vi "ATCcont.vi"() -> ()   [LabVIEW 2014]
doc: "ATC app"
panel:
  in  "정지":bool
  in  "피드백":bool
  in  "정보1":bool
  in  "도움말":bool
  in  "?":bool
  in  "?":bool
  in  "탭":T1(tab)
  in  "메모":string="필요한 메모를 할수 있습니다. "
  in  "SID&RadarVector. 2":string="SID&RadarVector. "
  in  "인사말":string="인사말"
  in  "CD관제기관":string="관제기관"
  in  "콜사인":string="콜사인\n콜사인\n콜사인"
  in  "도착공항":string="도착공항"
  in  "SID&RadarVector":string="SID&RadarVector"
  in  "비행고도":string="비행고도"
  in  "인사말2":string="인사말"
  in  "콜사인2":string="콜사인"
  in  "콜사인3":string="콜사인"
  in  "콜사인4":string="콜사인"
  in  "콜사인5":string="콜사인"
  in  "콜사인6":string="콜사인"
  in  "도착공항2":string="도착공항"
  in  "제한고도":string="제한고도"
  in  "비행고도2":string="비행고도"
  in  "D접속주파수":string="접속주파수"
  in  "스콱번호":string="스콱번호"
  in  "도착공항3":string="도착공항"
  in  "SID&RadarVector. 3":string="SID&RadarVector. "
  in  "제한고도2":string="제한고도"
  in  "비행고도3":string="비행고도"
  in  "D접속주파수2":string="접속주파수"
  in  "스콱번호2":string="스쾃번호"
  in  "콜사인7":string="콜사인"
  in  "콜사인8":string="콜사인"
  in  "G관제기관":string="관제기관"
  in  "G접속주파수2":string="접속주파수"
  in  "G관제기관2":string="관제기관"
  in  "G접속주파수":string="접속주파수"
  in  "콜사인9":string="콜사인"
  in  "유도로 2":string="유도로"
  in  "유도로":string="유도로"
  in  "방향 2":string="방향"
  in  "방향":string="방향"
  in  "메모2":string="필요한 메모를 할수 있습니다. "
  in  "T관제기관2":string="관제기관"
  in  "콜사인24":string="콜사인"
  in  "T접속주파수2":string="접속주파수"
  in  "T접속주파수":string="접속주파수"
  in  "T관제기관":string="관제기관"
  in  "콜사인23":string="콜사인"
  in  "활주로9":string="활주로"
  in  "G관제기관4":string="관제기관"
  in  "콜사인22":string="콜사인"
  in  "콜사인21":string="콜사인"
  in  "콜사인20":string="콜사인"
  in  "콜사인19":string="콜사인"
  in  "활주로8":string="활주로"
  in  "활주로7":string="활주로"
  in  "콜사인17":string="콜사인"
  in  "활주로6":string="활주로"
  in  "콜사인18":string="콜사인"
  in  "활주로5":string="활주로"
  in  "콜사인16":string="콜사인"
  in  "활주로4":string="활주로"
  in  "콜사인15":string="콜사인"
  in  "활주로3":string="활주로"
  in  "콜사인14":string="콜사인"
  in  "콜사인13":string="콜사인"
  in  "현재기압2":string="현재기압"
  in  "출발공항":string="출발공항"
  in  "활주로2":string="활주로"
  in  "현재기압":string="현재기압"
  in  "출발공항2":string="출발공항"
  in  "활주로1":string="활주로"
  in  "콜사인12":string="콜사인"
  in  "콜사인11":string="콜사인"
  in  "G관제기관3":string="관제기관"
  in  "인사3":string="인사"
  in  "콜사인34 2":string="콜사인"
  in  "D관제기관2":string="관제기관"
  in  "D관제기관":string="관제기관"
  in  "T관제기관3":string="관제기관"
  in  "메모3":string="필요한 메모를 할수 있습니다. "
  in  "인사4":string="인사"
  in  "콜사인25":string="콜사인"
  in  "활주로10":string="활주로"
  in  "콜사인26":string="콜사인"
  in  "바람방향":string="바람방향"
  in  "풍속":string="풍속"
  in  "콜사인28":string="콜사인"
  in  "활주로13":string="활주로"
  in  "콜사인29":string="콜사인"
  in  "활주로12":string="활주로"
  in  "콜사인30":string="콜사인"
  in  "활주로14":string="활주로"
  in  "콜사인31":string="콜사인"
  in  "활주로15":string="활주로"
  in  "T관제기관4":string="관제기관"
  in  "콜사인32":string="콜사인"
  in  "현재고도":string="현재고도"
  in  "허가고도":string="허가고도"
  in  "콜사인33":string="콜사인"
  in  "접속주파수":string="접속주파수"
  in  "콜사인34":string="콜사인"
  in  "접속주파수2":string="접속주파수"
  in  "순항고도or이니셜고도":string="순항고도or이니셜고도"
  in  "D관제기관5":string="관제기관"
  in  "메모 4":string="필요한 메모를 할수 있습니다. "
  in  "인사5":string="인사"
  in  "D관제기관3":string="관제기관"
  in  "콜사인35":string="콜사인"
  in  "현재고도A":string="현재고도"
  in  "콜사인36":string="콜사인"
  in  "D관제기관4":string="관제기관"
  in  "허가고도4":string="허가고도"
  in  "허가고도5":string="허가고도"
  in  "콜사인37":string="콜사인"
  in  "콜사인38":string="콜사인"
  in  "허가고도6":string="허가고도"
  in  "허가고도7":string="허가고도"
  in  "콜사인39":string="콜사인"
  in  "콜사인40":string="콜사인"
  in  "C관제기관":string="관제기관"
  in  "A접속주파수":string="접속주파수"
  in  "C관제기관2":string="관제기관"
  in  "A접속주파수2":string="접속주파수"
  in  "콜사인41":string="콜사인"
  in  "콜사인38 2":string="콜사인"
  in  "D관제기관6":string="관제기관"
  in  "허가고도6 2":string="허가고도"
  in  "허가고도6 3":string="허가고도"
  in  "콜사인39 2":string="콜사인"
  in  "메모5":string="필요한 메모를 할수 있습니다. "
  in  "인사말 2":string="인사말"
  in  "허가고도 2":string="허가고도"
  in  "지점":string="지점"
  in  "허가고도7 2":string="허가고도"
  in  "콜사인38 3":string="콜사인"
  in  "콜사인39 3":string="콜사인"
  in  "허가고도7 3":string="허가고도"
  in  "지점 2":string="지점"
  in  "메모6":string="필요한 메모를 할수 있습니다. "
  in  "A관제기관3":string="관제기관"
  in  "콜사인46":string="콜사인"
  in  "날시정보":string="날시정보"
  in  "고도":string="고도"
  in  "콜사인47":string="콜사인"
  in  "A관제기관4":string="관제기관"
  in  "L활주로":string="활주로"
  in  "도착공항4":string="도착공항"
  in  "현재기압":string="현재기압"
  in  "콜사인48":string="콜사인"
  in  "A관제기관5":string="관제기관"
  in  "L활주로":string="활주로"
  in  "도착공항5":string="도착공항"
  in  "현재기압":string="현재기압"
  in  "콜사인49":string="콜사인"
  in  "고도":string="고도"
  in  "콜사인50":string="콜사인"
  in  "고도":string="고도"
  in  "콜사인51":string="콜사인"
  in  "고도":string="고도"
  in  "고도":string="고도"
  in  "콜사인52":string="콜사인"
  in  "콜사인53":string="콜사인"
  in  "A관제기관":string="관제기관"
  in  "풍속":string="풍속"
  in  "바람방향":string="바람방향"
  in  "L활주로3":string="활주로"
  in  "콜사인54":string="콜사인"
  in  "L활주로":string="활주로"
  in  "콜사인55":string="콜사인"
  in  "A관제기관2":string="관제기관"
  in  "L활주로":string="활주로"
  in  "ILS":string="주파수(ils)"
  in  "콜사인56":string="콜사인"
  in  "L활주로6":string="활주로"
  in  "ILS2":string="주파수(ils)"
  in  "콜사인57":string="콜사인"
  in  "T관제기관":string="관제기관"
  in  "T접속주파수":string="접속주파수"
  in  "콜사인58":string="콜사인"
  in  "콜사인59":string="콜사인"
  in  "관제기관":string="관제기관"
  in  "T접속주파수":string="접속주파수"
  in  "메모7":string="필요한 메모를 할수 있습니다. "
  in  "바람방향":string="바람방향"
  in  "관제기관":string="관제기관"
  in  "콜사인60":string="콜사인"
  in  "L활주로7":string="활주로"
  in  "콜사인61":string="콜사인"
  in  "풍속":string="풍속"
  in  "콜사인62":string="콜사인"
  in  "L활주로":string="활주로"
  in  "L활주로":string="활주로"
  in  "관제기관":string="관제기관"
  in  "콜사인63":string="콜사인"
  in  "관제기관3":string="관제기관"
  in  "콜사인64":string="콜사인"
  in  "L활주로":string="활주로"
  in  "G관제기관":string="관제기관"
  in  "G접속주파수":string="접속주파수"
  in  "콜사인65":string="콜사인"
  in  "관제기관":string="관제기관"
  in  "G접속주파수":string="접속주파수"
  in  "콜사인70":string="콜사인"
  in  "C활주로3":string="활주로"
  in  "C활주로2":string="활주로"
  in  "관제기관3 2":string="관제기관"
  in  "C활주로":string="활주로"
  in  "콜사인69":string="콜사인"
  in  "관제기관2":string="관제기관"
  in  "메모8":string="필요한 메모를 할수 있습니다. "
  in  "관제기관":string="관제기관"
  in  "콜사인66":string="콜사인"
  in  "콜사인67":string="콜사인"
  in  "게이트번호":string="게이트번호"
  in  "THEN":string="then"
  in  "콜사인68":string="콜사인"
  in  "게이트번호2":string="게이트번호"
  in  "THEN2":string="then"
  in  "콜사인10":string="콜사인"
  in  "관제기관4":string="관제기관"
  in  "콜사인71":string="콜사인"
  in  "콜사인72":string="콜사인"
  # "ver.3.0.0.55"
  # "~"
  # "Good"
  # "Clearance Delivery"
  # "Pilot"
  # "at FL"
  # "Request IFR Clearance to"
  # "Airport via"
  # "~"
  # "Good"
  # "Controller"
  # ",  Clearance  Delivery, standby."
  # "Pilot"
  # "Stand by,"
  # "Controller"
  # "Delivery 또는 Delivery, Are you ready to copy?"
  # "Pilot"
  # "Go Ahead 또는 Ready to copy"
  # "Airport via"
  # ", Cleared to"
  # "Controller"
  # "ft expect FL"
  # "then as filed. Climb and Maintain"
  # "Departure Frequency"
  # "Read back."
  # "Squawk"
  # "Pilot"
  # "Airport via"
  # "Cleared to"
  # ","
  # "then as filed."
  # "Climb and Maintain"
  # "ft expect FL"
  # "Departure Frequency"
  # "and  Squawk"
  # "Controller"
  # ", Read back is corrent contact"
  # "Ground"
  # "bye bye~."
  # "Pilot"
  # "Roger, contact"
  # ", bye bye~"
  # "Pilot"
  # "Good"
  # "~"
  # "ready for push back and Engine Start."
  # ","
  # ", Rwy"
  # "Push Back and Engine Start Approved, heading to"
  # "Controller"
  # ","
  # "QNH"
  # "Read Back."
  # "Pilot"
  # "Roger\nPush Back and Engine Start Approved, heading to"
  # ", Rwy"
  # "QNH"
  # "Ready for taxi to the Rwy"
  # ","
  # "Pilot"
  # "- Push back 완료 후 -"
  # ", Ready for Taxi to Rwy"
  # "Controller"
  # ", taxi to"
  # "via taxiway"
  # ", Roger"
  # "Pilot"
  # "via taxiway"
  # "Taxi to"
  # "- 활주로를 건널 상황일 때 -"
  # "Pilot"
  # "Request Cross Rwy"
  # "Controller"
  # ", cleared Cross Rwy"
  # "Pilot"
  # "cleared Cross Rwy"
  # "Controller"
  # "Squawk Mode C."
  # "Pilot"
  # ", Roger squawk mode 'C'"
  # "------------------------ 홀딩 포인트 도착 후 ----------------------------------"
  # "Pilot"
  # "hold short of Rwy"
  # ","
  # "Controller"
  # "Roger,"
  # "contact"
  # "Tower"
  # "bye bye~"
  # "Pilot"
  # "Contact"
  # "Pilot"
  # "Good"
  # "~"
  # ",  hold short Rwy"
  # ", Ready for Departure"
  # "(곧바로 이륙허가)"
  # "Controller"
  # ", wind"
  # "knot, cleared for take off."
  # "at"
  # "(활주로 정렬대기)"
  # "Controller"
  # "Line up and wait Rwy"
  # "Pilot"
  # "Line up and wait Rwy"
  # "Roger,"
  # "(홀딩 포인트에서 대기)"
  # "Controller"
  # ", Hold short rwy"
  # ","
  # "Pilot"
  # "Hold short of Rwy"
  # "Roger,"
  # "- 이 륙 후 -"
  # "Pilot"
  # "ft."
  # "Airborn Passing"
  # "ft, Climbing"
  # ","
  # "Controller"
  # ", contact"
  # "Departure,"
  # "bye bye~"
  # "Pilot"
  # ", Roger"
  # "Contact"
  # "Departure,"
  # "bye bye~"
  # "Good"
  # "~"
  # "Pilot"
  # "Passing"
  # "expect"
  # "with (SID)."
  # ","
  # ","
  # "Controller"
  # "Departure, Radar Contact, Climb via (SID) to"
  # ","
  # "."
  # "Pilot"
  # "Roger, Climb via"
  # ","
  # "-고도제한 해제시-"
  # "Controller"
  # "Departure, Radar Contact, Climb via (SID) to"
  # ", Cancel Level Restrictions."
  # "Pilot"
  # "Roger, Climb via (SID) to"
  # ", Cancel Level Restrictions,"
  # "-속도제한 해제시-"
  # "Controller"
  # "Departure, Radar Contact, Climb via (SID) to"
  # ", Cancel Speed Restrictions."
  # "Pilot"
  # "Roger, Climb via (SID) to"
  # ", Cancel Speed Restrictions,"
  # "Controller"
  # "Control,"
  # ", bye bye."
  # ", You are leaving my airspace, Contact"
  # "Pilot"
  # "Contact"
  # "G'day"
  # "Control,"
  # ","
  # "Pilot"
  # "Good"
  # "Decend and maintain FL"
  # "with (SID)."
  # "-하강 발부-"
  # "Controller"
  # "by"
  # ", Descend and Maintain"
  # "Pilot"
  # "Descend and Maintain"
  # "by"
  # "Pilot"
  # ","
  # "FL"
  # "with information"
  # ","
  # ", Expect vector to ILS Rwy"
  # "approach"
  # "Controller"
  # "QNH"
  # "Roger,"
  # "Pilot"
  # ", Expect vector to ILS Rwy"
  # "final approach"
  # "QNH"
  # "Controller"
  # ", Decend and maintain FL"
  # "Pilot"
  # "Decend and maintain FL"
  # "Roger,"
  # "Controller"
  # ", Decend and maintain"
  # "ft"
  # "Pilot"
  # "Roger"
  # "Decend and maintain"
  # "ft"
  # "Controller"
  # ","
  # "for landing"
  # "wind"
  # "knots active Rwy"
  # "at"
  # "Pilot"
  # "Roger,"
  # "Rwy"
  # "for landing"
  # "Controller"
  # ","
  # "approach use Rwy"
  # "ILS"
  # "Roger,"
  # "Pilot"
  # "Use Rwy"
  # "ILS"
  # "- 정 렬 후 -"
  # "Pilot"
  # "Approach,"
  # ", Established on Localizer."
  # "Controller"
  # "Tower,"
  # "Good day,"
  # "Roger, Contact"
  # "Pilot"
  # "Contact"
  # "Tower"
  # "Good day,"
  # "Pilot"
  # ","
  # "Inbound Approaching Rwy"
  # "Controller"
  # ", Wind"
  # "at"
  # "knots Rwy"
  # ", Cleared to land"
  # "Pilot"
  # "Rwy"
  # "Cleared to land"
  # "Pilot"
  # ","
  # "- 착 륙 후 -"
  # ","
  # "Pilot"
  # "Touch down with Rwy"
  # "Controller"
  # "Roger, change squawk mode Standby and contact"
  # "bye bye~"
  # "ground"
  # "Pilot"
  # ", Roger"
  # "bye bye~"
  # "Change squawk mode standby and contact"
  # "- 활주로를 건널 상황일 때 -"
  # "Pilot"
  # ","
  # "Request Cross Rwy"
  # "Controller"
  # ", Cross Rwy"
  # "approved."
  # "Pilot"
  # "Cross Rwy"
  # "approved"
  # ","
  # "Pilot"
  # "Ready to taxi to the Gate"
  # "Controller"
  # ", taxi to the gate"
  # "via taxi way"
  # "Roger,"
  # "Pilot"
  # "taxi to the gate"
  # "via taxi way"
  # "- 게이트 도착 후 -"
  # "Pilot"
  # "at Gate and Engine Shut down."
  # "Thank you for your ATC service."
  # "Controller"
  # ", at the gate and Engine Shut down, Thank you ~~"
  # "Pilot"
  # "Have a nice day,"
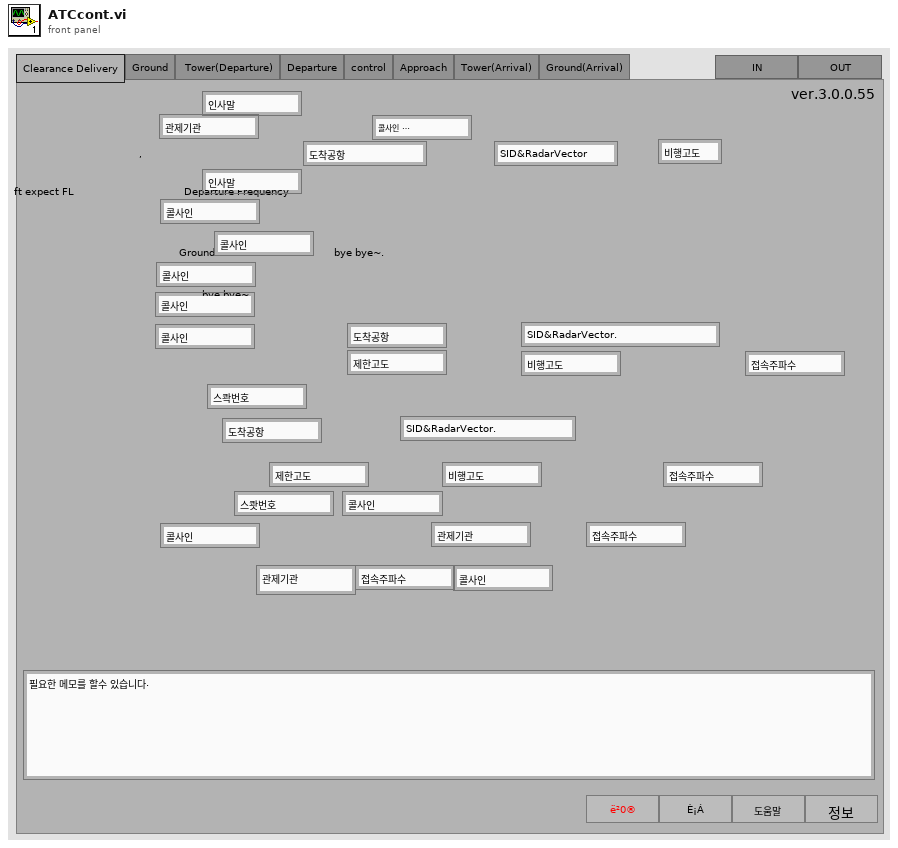
[diagram p1: front panel]
types:
  T1 = enum32{"Clearance Delivery", "Ground", " Tower(Departure)", "Departure", "control", "Approach", "Tower(Arrival)", "Ground(Arrival)"}
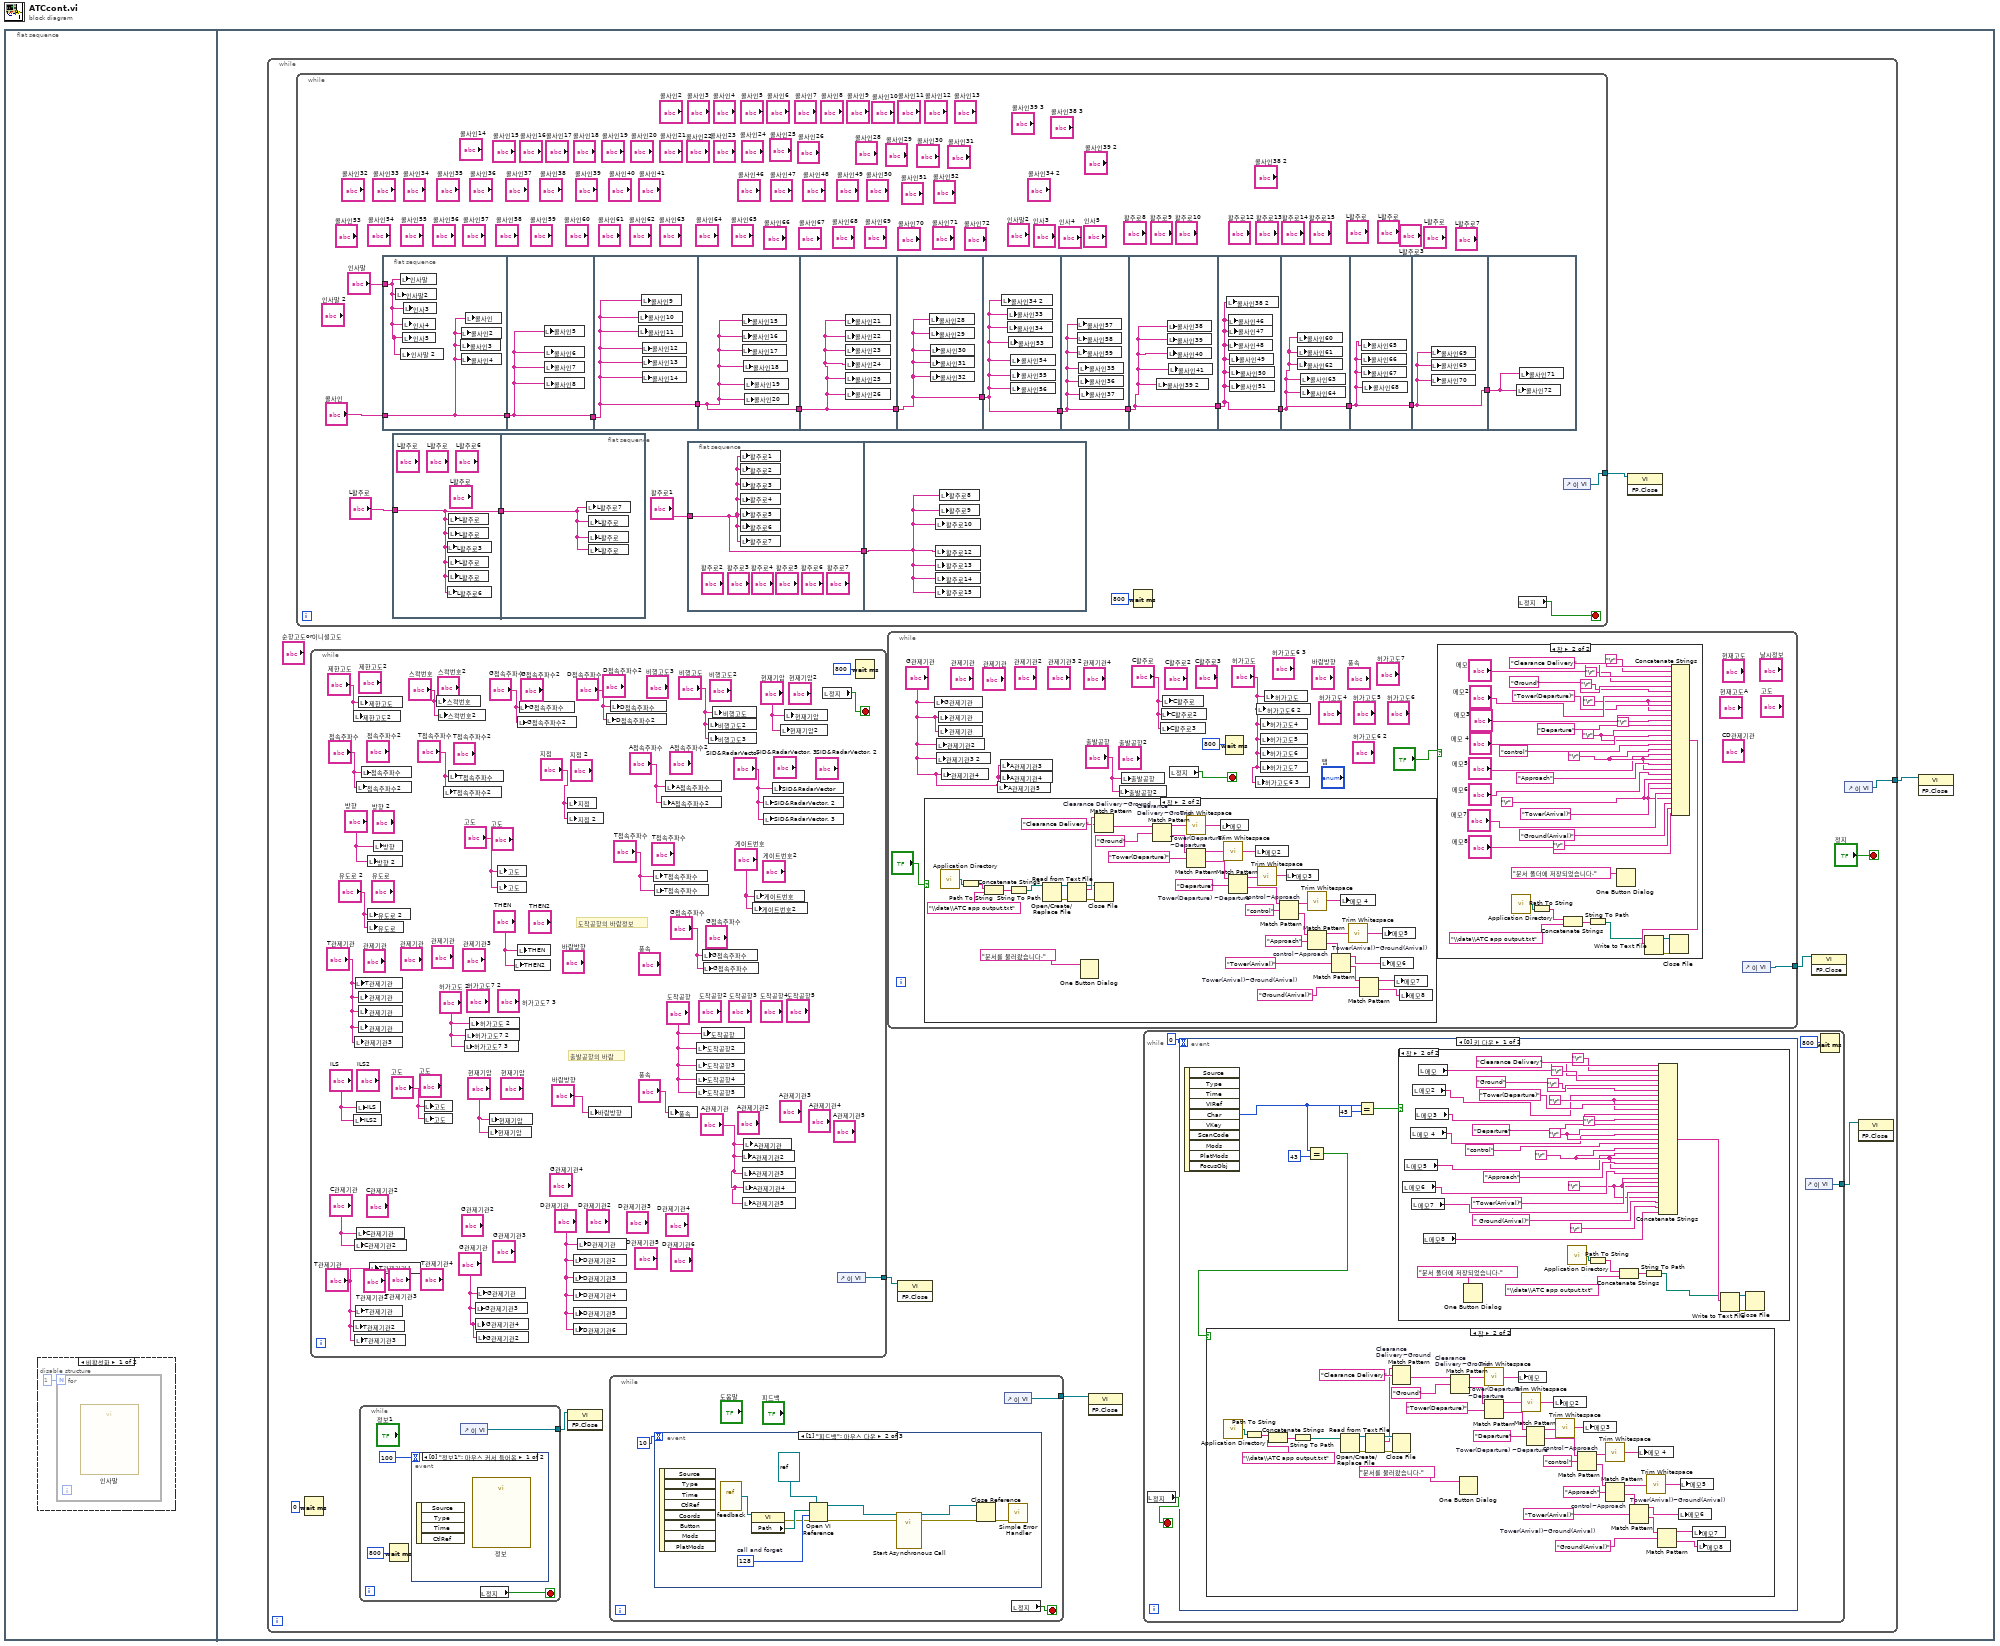
[diagram p0: block diagram]
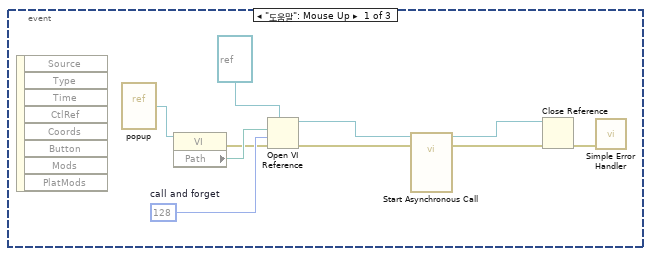
[diagram p3: hidden frame]
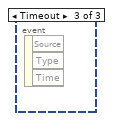
[diagram p4: hidden frame]
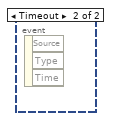
[diagram p7: hidden frame]
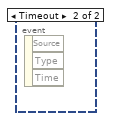
[diagram p8: hidden frame]
diagram:
  n1 = flat-sequence {
    frame #0 {
      n2 = disable-structure shown="비활성화" {
        frame Disabled {
          n3 = for {
            N: 1 -> [_]
            n4 = call "인사말"() -> ()  [unwired: 10 in, 2 out]
          }
        }
        frame Enabled {
        }
      }
    }
    frame #1 {
      n5 = while {
        tunnel: [w3] -> w2
        stop <- "정지" stop-if-true
        n6 = while {
          tunnel: [w122] -> w7
          stop <- w121 stop-if-true
          n7 = flat-sequence {
            tunnel: [w144] -> w140
            tunnel: "콜사인" -> [w144]
            tunnel: "인사말" -> [w143]
            tunnel: w140 -> [w145]
            tunnel: [w145] -> w139
            tunnel: w139 -> [w146]
            tunnel: [w146] -> w138
            tunnel: w138 -> [w147]
            tunnel: [w147] -> w137
            tunnel: [w148] -> w136
            tunnel: w137 -> [w148]
            tunnel: w136 -> [w149]
            tunnel: [w149] -> w135
            tunnel: [w150] -> w134
            tunnel: w135 -> [w150]
            tunnel: w134 -> [w151]
            tunnel: [w151] -> w133
            tunnel: w133 -> [w152]
            tunnel: [w152] -> w132
            tunnel: w132 -> [w153]
            tunnel: [w153] -> w131
            tunnel: w131 -> [w154]
            tunnel: [w154] -> w130
            tunnel: w130 -> [w155]
            tunnel: [w155] -> w129
            tunnel: w129 -> [w156]
            tunnel: [w156] -> w128
            tunnel: w128 -> [w157]
            frame #0 {
              n8 = local write "인사말2"(w143) -> ()
              n9 = local write "인사말"(w143) -> ()
              n10 = local write "인사말 2"(w143) -> ()
              n11 = local write "인사4"(w143) -> ()
              n12 = local write "인사5"(w143) -> ()
              n13 = local write "인사3"(w143) -> ()
              n14 = local write "콜사인3"(w144) -> ()
              n15 = local write "콜사인2"(w144) -> ()
              n16 = local write "콜사인4"(w144) -> ()
              n17 = local write "콜사인"(w144) -> ()
            }
            frame #1 {
              n18 = local write "콜사인5"(w145) -> ()
              n19 = local write "콜사인6"(w145) -> ()
              n20 = local write "콜사인7"(w145) -> ()
              n21 = local write "콜사인8"(w145) -> ()
            }
            frame #2 {
              n22 = local write "콜사인10"(w146) -> ()
              n23 = local write "콜사인11"(w146) -> ()
              n24 = local write "콜사인9"(w146) -> ()
              n25 = local write "콜사인12"(w146) -> ()
              n26 = local write "콜사인13"(w146) -> ()
              n27 = local write "콜사인14"(w146) -> ()
            }
            frame #3 {
              n28 = local write "콜사인15"(w147) -> ()
              n29 = local write "콜사인16"(w147) -> ()
              n30 = local write "콜사인17"(w147) -> ()
              n31 = local write "콜사인18"(w147) -> ()
              n32 = local write "콜사인19"(w147) -> ()
              n33 = local write "콜사인20"(w147) -> ()
            }
            frame #4 {
              n34 = local write "콜사인21"(w148) -> ()
              n35 = local write "콜사인22"(w148) -> ()
              n36 = local write "콜사인23"(w148) -> ()
              n37 = local write "콜사인24"(w148) -> ()
              n38 = local write "콜사인25"(w148) -> ()
              n39 = local write "콜사인26"(w148) -> ()
            }
            frame #5 {
              n40 = local write "콜사인28"(w149) -> ()
              n41 = local write "콜사인29"(w149) -> ()
              n42 = local write "콜사인30"(w149) -> ()
              n43 = local write "콜사인31"(w149) -> ()
              n44 = local write "콜사인32"(w149) -> ()
            }
            frame #6 {
              n45 = local write "콜사인34 2"(w150) -> ()
              n46 = local write "콜사인33"(w150) -> ()
              n47 = local write "콜사인34"(w150) -> ()
              n48 = local write "콜사인53"(w150) -> ()
              n49 = local write "콜사인54"(w150) -> ()
              n50 = local write "콜사인55"(w150) -> ()
              n51 = local write "콜사인56"(w150) -> ()
            }
            frame #7 {
              n52 = local write "콜사인57"(w151) -> ()
              n53 = local write "콜사인58"(w151) -> ()
              n54 = local write "콜사인59"(w151) -> ()
              n55 = local write "콜사인35"(w151) -> ()
              n56 = local write "콜사인36"(w151) -> ()
              n57 = local write "콜사인37"(w151) -> ()
            }
            frame #8 {
              n58 = local write "콜사인39 2"(w152) -> ()
              n59 = local write "콜사인38"(w152) -> ()
              n60 = local write "콜사인39"(w152) -> ()
              n61 = local write "콜사인40"(w152) -> ()
              n62 = local write "콜사인41"(w152) -> ()
            }
            frame #9 {
              n63 = local write "콜사인38 2"(w153) -> ()
              n64 = local write "콜사인46"(w153) -> ()
              n65 = local write "콜사인47"(w153) -> ()
              n66 = local write "콜사인48"(w153) -> ()
              n67 = local write "콜사인49"(w153) -> ()
              n68 = local write "콜사인50"(w153) -> ()
              n69 = local write "콜사인51"(w153) -> ()
            }
            frame #10 {
              n70 = local write "콜사인60"(w154) -> ()
              n71 = local write "콜사인61"(w154) -> ()
              n72 = local write "콜사인62"(w154) -> ()
              n73 = local write "콜사인63"(w154) -> ()
              n74 = local write "콜사인64"(w154) -> ()
            }
            frame #11 {
              n75 = local write "콜사인65"(w155) -> ()
              n76 = local write "콜사인66"(w155) -> ()
              n77 = local write "콜사인67"(w155) -> ()
              n78 = local write "콜사인68"(w155) -> ()
            }
            frame #12 {
              n79 = local write "콜사인69"(w156) -> ()
              n80 = local write "콜사인69"(w156) -> ()
              n81 = local write "콜사인70"(w156) -> ()
            }
            frame #13 {
              n82 = local write "콜사인72"(w157) -> ()
              n83 = local write "콜사인71"(w157) -> ()
            }
          }
          n84 = flat-sequence {
            tunnel: "L활주로" -> [w160]
            tunnel: [w160] -> w142
            tunnel: w142 -> [w161]
            frame #0 {
              n85 = local write "L활주로3"(w160) -> ()
              n86 = local write "L활주로6"(w160) -> ()
              n87 = local write "L활주로"(w160) -> ()
              n88 = local write "L활주로"(w160) -> ()
              n89 = local write "L활주로"(w160) -> ()
              n90 = local write "L활주로"(w160) -> ()
            }
            frame #1 {
              n91 = local write "L활주로7"(w161) -> ()
              n92 = local write "L활주로"(w161) -> ()
              n93 = local write "L활주로"(w161) -> ()
              n94 = local write "L활주로"(w161) -> ()
            }
          }
          n95 = flat-sequence {
            tunnel: [w158] -> w141
            tunnel: "활주로1" -> [w158]
            tunnel: w141 -> [w159]
            frame #0 {
              n96 = local write "활주로1"(w158) -> ()
              n97 = local write "활주로2"(w158) -> ()
              n98 = local write "활주로3"(w158) -> ()
              n99 = local write "활주로4"(w158) -> ()
              n100 = local write "활주로5"(w158) -> ()
              n101 = local write "활주로6"(w158) -> ()
              n102 = local write "활주로7"(w158) -> ()
            }
            frame #1 {
              n103 = local write "활주로10"(w159) -> ()
              n104 = local write "활주로12"(w159) -> ()
              n105 = local write "활주로13"(w159) -> ()
              n106 = local write "활주로14"(w159) -> ()
              n107 = local write "활주로15"(w159) -> ()
              n108 = local write "활주로8"(w159) -> ()
              n109 = local write "활주로9"(w159) -> ()
            }
          }
          n110 = Wait (ms)(milliseconds to wait=u32 800 ("대기 시간(ms)")) -> ()  [unwired: 1 out]
          n111 = local read "정지"() -> (w121:bool)
          n112 = control-ref of="이 VI"() -> (w122:refnum<vi>)
        }
        n113 = Wait (ms)(milliseconds to wait=u32 0 ("대기 시간(ms)")) -> ()  [unwired: 1 out]
        n114 = while {
          tunnel: [w245] -> w10
          stop <- w244 stop-if-true
          # "출발공항의 바람"
          # "도착공항의 바람정보"
          n115 = local write "제한고도2"("제한고도") -> ()
          n116 = local write "T관제기관2"("T관제기관") -> ()
          n117 = local write "ILS2"("ILS") -> ()
          n118 = local write "관제기관3"("T관제기관") -> ()
          n119 = local write "C관제기관2"("C관제기관") -> ()
          n120 = local write "T관제기관3"("T관제기관") -> ()
          n121 = local write "T관제기관"("T관제기관") -> ()
          n122 = local write "T관제기관"("T관제기관") -> ()
          n123 = local write "C관제기관"("C관제기관") -> ()
          n124 = local write "접속주파수2"("접속주파수") -> ()
          n125 = local write "ILS"("ILS") -> ()
          n126 = local write "제한고도"("제한고도") -> ()
          n127 = local write "관제기관"("T관제기관") -> ()
          n128 = local write "관제기관"("T관제기관") -> ()
          n129 = local write "관제기관"("T관제기관") -> ()
          n130 = local write "접속주파수"("접속주파수") -> ()
          n131 = local write "방향 2"("방향") -> ()
          n132 = local write "유도로 2"("유도로 2") -> ()
          n133 = local write "유도로"("유도로 2") -> ()
          n134 = local write "T관제기관4"("T관제기관") -> ()
          n135 = local write "방향"("방향") -> ()
          n136 = local write "고도"("고도") -> ()
          n137 = local write "고도"("고도") -> ()
          n138 = local write "스콱번호"("스콱번호") -> ()
          n139 = local write "스콱번호2"("스콱번호") -> ()
          n140 = local write "T접속주파수2"("T접속주파수") -> ()
          n141 = local write "T접속주파수"("T접속주파수") -> ()
          n142 = local write "허가고도7 3"("허가고도 2") -> ()
          n143 = local write "허가고도7 2"("허가고도 2") -> ()
          n144 = local write "허가고도 2"("허가고도 2") -> ()
          n145 = local write "G관제기관3"("G관제기관") -> ()
          n146 = local write "G관제기관4"("G관제기관") -> ()
          n147 = local write "G관제기관2"("G관제기관") -> ()
          n148 = local write "G관제기관"("G관제기관") -> ()
          n149 = local write "현재기압"("현재기압") -> ()
          n150 = local write "현재기압"("현재기압") -> ()
          n151 = local write "고도"("고도") -> ()
          n152 = local write "고도"("고도") -> ()
          n153 = local write "THEN2"("THEN") -> ()
          n154 = local write "G접속주파수2"("G접속주파수") -> ()
          n155 = local write "THEN"("THEN") -> ()
          n156 = local write "G접속주파수"("G접속주파수") -> ()
          n157 = local write "지점"("지점") -> ()
          n158 = local write "지점 2"("지점") -> ()
          n159 = local write "D관제기관2"("D관제기관") -> ()
          n160 = local write "D관제기관3"("D관제기관") -> ()
          n161 = local write "D관제기관4"("D관제기관") -> ()
          n162 = local write "D관제기관5"("D관제기관") -> ()
          n163 = local write "D관제기관6"("D관제기관") -> ()
          n164 = local write "D관제기관"("D관제기관") -> ()
          n165 = local write "바람방향"("바람방향") -> ()
          n166 = local write "D접속주파수2"("D접속주파수") -> ()
          n167 = local write "D접속주파수"("D접속주파수") -> ()
          n168 = local write "T접속주파수"("T접속주파수") -> ()
          n169 = local write "T접속주파수"("T접속주파수") -> ()
          n170 = local write "A접속주파수2"("A접속주파수") -> ()
          n171 = local write "A접속주파수"("A접속주파수") -> ()
          n172 = local write "풍속"("풍속") -> ()
          n173 = local write "도착공항2"("도착공항") -> ()
          n174 = local write "도착공항3"("도착공항") -> ()
          n175 = local write "도착공항4"("도착공항") -> ()
          n176 = local write "도착공항5"("도착공항") -> ()
          n177 = local write "도착공항"("도착공항") -> ()
          n178 = local write "G접속주파수"("G접속주파수") -> ()
          n179 = local write "G접속주파수"("G접속주파수") -> ()
          n180 = local write "비행고도2"("비행고도") -> ()
          n181 = local write "비행고도3"("비행고도") -> ()
          n182 = local write "비행고도"("비행고도") -> ()
          n183 = local write "A관제기관2"("A관제기관") -> ()
          n184 = local write "A관제기관3"("A관제기관") -> ()
          n185 = local write "A관제기관5"("A관제기관") -> ()
          n186 = local write "A관제기관4"("A관제기관") -> ()
          n187 = local write "A관제기관"("A관제기관") -> ()
          n188 = local write "게이트번호2"("게이트번호") -> ()
          n189 = local write "게이트번호"("게이트번호") -> ()
          n190 = local write "SID&RadarVector. 2"("SID&RadarVector") -> ()
          n191 = local write "SID&RadarVector. 3"("SID&RadarVector") -> ()
          n192 = local write "SID&RadarVector"("SID&RadarVector") -> ()
          n193 = local write "현재기압2"("현재기압") -> ()
          n194 = local write "현재기압"("현재기압") -> ()
          n195 = local read "정지"() -> (w244:bool)
          n196 = control-ref of="이 VI"() -> (w245:refnum<vi>)
          n197 = Wait (ms)(milliseconds to wait=u32 800 ("대기 시간(ms)")) -> ()  [unwired: 1 out]
        }
        n198 = while {
          tunnel: [w118] -> w8
          stop <- w117 stop-if-true
          n199 = Wait (ms)(milliseconds to wait=u32 800 ("대기 시간(ms)")) -> ()  [unwired: 1 out]
          n200 = event shown="[0] \"정보1\": 마우스 커서 들어옴" {
            selector: _ -> [_ _]
            dyn-events: _ -> [_ _]
            timeout: 100 -> [_ _]
            event "정보1": Mouse Enter {
              n201 = event-data() -> ()  [unwired: 1 in, 4 out]
              n202 = call "정보"() -> ()  [unwired: 10 in, 2 out]
            }
            event Timeout {
              n203 = event-data() -> ()  [unwired: 1 in, 3 out]
            }
          }
          n204 = control-ref of="이 VI"() -> (w118:refnum<vi>)
          n205 = local read "정지"() -> (w117:bool)
        }
        n206 = invoke class="VI" method="FP.Close"(reference=w8) -> ()  [unwired: 2 in, 3 out]
        n207 = while {
          tunnel: [w13] -> w9
          stop <- w12 stop-if-true
          n208 = event shown="[1] \"피드백\": 마우스 다운" {
            selector: _ -> [_ _ _]
            dyn-events: _ -> [_ _ _]
            timeout: 10 -> [_ _ _]
            event "도움말": Mouse Up {
              w24 = 128  # call and forget
              n209 = event-data() -> ()  [unwired: 1 in, 8 out]
              n210 = vi-ref "popup.vi"() -> (w17:refnum<vi>)
              n211 = property class="VI"(reference=w17) -> (error out=w18:errorcluster, "Path"=w19:path)  [unwired: 1 in, 1 out]
              n212 = Open VI Reference(type specifier VI Refnum (for type only)=refnum<vi> refnum, vi path=w19, options=w24, error in (no error)=w18) -> (vi reference=w16:refnum<vi>, error out=w22:errorcluster)  [unwired: 2 in]
              n213 = call-by-ref "Start Asynchronous Call"(reference=w16, error in=w22) -> (reference out=w15:refnum<vi>, error out=w21:errorcluster)  [unwired: 12 in]
              n214 = Close Reference(reference=w15, error in (no error)=w21) -> (error out=w20:errorcluster)
              n215 = call <vilib>:"Simple Error Handler.vi"("error in (no error)"=w20) -> ()  [unwired: 4 in, 5 out]
            }
            event "피드백": Mouse Down {
              w34 = 128  # call and forget
              n216 = event-data() -> ()  [unwired: 1 in, 8 out]
              n217 = vi-ref "feedback.vi"() -> (w27:refnum<vi>)
              n218 = property class="VI"(reference=w27) -> (error out=w28:errorcluster, "Path"=w29:path)  [unwired: 1 in, 1 out]
              n219 = Open VI Reference(type specifier VI Refnum (for type only)=refnum<vi> refnum, vi path=w29, options=w34, error in (no error)=w28) -> (vi reference=w26:refnum<vi>, error out=w32:errorcluster)  [unwired: 2 in]
              n220 = call-by-ref "Start Asynchronous Call"(reference=w26, error in=w32) -> (reference out=w25:refnum<vi>, error out=w31:errorcluster)  [unwired: 12 in]
              n221 = Close Reference(reference=w25, error in (no error)=w31) -> (error out=w30:errorcluster)
              n222 = call <vilib>:"Simple Error Handler.vi"("error in (no error)"=w30) -> ()  [unwired: 4 in, 5 out]
            }
            event Timeout {
              n223 = event-data() -> ()  [unwired: 1 in, 3 out]
            }
          }
          n224 = control-ref of="이 VI"() -> (w13:refnum<vi>)
          n225 = local read "정지"() -> (w12:bool)
        }
        n226 = while {
          tunnel: [w162] -> w6
          stop <- w163 stop-if-true
          n227 = case shown="참" "?" {
            frame False {
            }
            frame True {
              n228 = call <vilib>:"Application Directory.vi"() -> ("Application Directory"=w175:path)
              n229 = Path To String(path=w175) -> (string=w173:string)
              n230 = Concatenate Strings(w173, "\\data\\ATC app output.txt" ("문자열")) -> (w172:string)
              n231 = String To Path(string=w172) -> (path=w171:path)
              n232 = Open/Create/Replace File(file path (use dialog)=w171) -> (refnum out=w189:refnum<file>, error out=w190:errorcluster)  [unwired: 5 in, 1 out]
              n233 = Read from Text File(file (use dialog)=w189, error in=w190) -> (refnum out=w191:refnum<file>, text=w197:string, error out=w192:errorcluster)  [unwired: 2 in, 1 out]
              n234 = One Button Dialog(message="문서를 불러왔습니다." ("메시지")) -> ()  [unwired: 1 in, 1 out]
              n235 = Match Pattern "Clearance Delivery~Ground"(string=w197, regular expression="Clearance Delivery" ("정규식")) -> (after substring=w194:string)  [unwired: 1 in, 3 out]
              n236 = Close File(refnum=w191, error in=w192) -> ()  [unwired: 2 out]
              n237 = Match Pattern "Clearance Delivery~Ground"(string=w194, regular expression="Ground" ("정규식")) -> (before substring=w199:string, after substring=w198:string)  [unwired: 1 in, 2 out]
              n238 = call <vilib>:"Trim Whitespace.vi"("string"=w199) -> ("trimmed string"=w188:string)  [unwired: 1 in]
              n239 = Match Pattern "Tower(Departure) ~Departure"(string=w198, regular expression="Tower(Departure)" ("정규식")) -> (before substring=w200:string, after substring=w203:string)  [unwired: 1 in, 2 out]
              n240 = local write "메모"(w188) -> ()
              n241 = call <vilib>:"Trim Whitespace.vi"("string"=w200) -> ("trimmed string"=w187:string)  [unwired: 1 in]
              n242 = Match Pattern "Tower(Departure) ~Departure"(string=w203, regular expression="Departure" ("정규식")) -> (before substring=w202:string, after substring=w209:string)  [unwired: 1 in, 2 out]
              n243 = local write "메모2"(w187) -> ()
              n244 = call <vilib>:"Trim Whitespace.vi"("string"=w202) -> ("trimmed string"=w186:string)  [unwired: 1 in]
              n245 = Match Pattern "control~Approach"(string=w209, regular expression="control" ("정규식")) -> (before substring=w207:string, after substring=w205:string)  [unwired: 1 in, 2 out]
              n246 = local write "메모3"(w186) -> ()
              n247 = call <vilib>:"Trim Whitespace.vi"("string"=w207) -> ("trimmed string"=w185:string)  [unwired: 1 in]
              n248 = Match Pattern "control~Approach"(string=w205, regular expression="Approach" ("정규식")) -> (before substring=w208:string, after substring=w182:string)  [unwired: 1 in, 2 out]
              n249 = Match Pattern "Tower(Arrival)~Ground(Arrival)"(string=w182, regular expression="Tower(Arrival)" ("정규식")) -> (before substring=w180:string, after substring=w178:string)  [unwired: 1 in, 2 out]
              n250 = local write "메모 4"(w185) -> ()
              n251 = call <vilib>:"Trim Whitespace.vi"("string"=w208) -> ("trimmed string"=w184:string)  [unwired: 1 in]
              n252 = Match Pattern "Tower(Arrival)~Ground(Arrival)"(string=w178, regular expression="Ground(Arrival)" ("정규식")) -> (before substring=w177:string, after substring=w176:string)  [unwired: 1 in, 2 out]
              n253 = local write "메모6"(w180) -> ()
              n254 = local write "메모5"(w184) -> ()
              n255 = local write "메모7"(w177) -> ()
              n256 = local write "메모8"(w176) -> ()
            }
          }
          n257 = local write "G관제기관"("G관제기관") -> ()
          n258 = local write "관제기관3 2"("G관제기관") -> ()
          n259 = local write "관제기관2"("G관제기관") -> ()
          n260 = local write "관제기관"("G관제기관") -> ()
          n261 = local write "관제기관"("G관제기관") -> ()
          n262 = local write "관제기관4"("G관제기관") -> ()
          n263 = local write "A관제기관5"("G관제기관") -> ()
          n264 = local write "A관제기관3"("G관제기관") -> ()
          n265 = local write "A관제기관4"("G관제기관") -> ()
          n266 = local write "출발공항2"("출발공항") -> ()
          n267 = local write "출발공항"("출발공항") -> ()
          n268 = local write "C활주로3"("C활주로") -> ()
          n269 = local write "C활주로2"("C활주로") -> ()
          n270 = local write "C활주로"("C활주로") -> ()
          n271 = local read "정지"() -> (w163:bool)
          n272 = Wait (ms)(milliseconds to wait=u32 800 ("대기 시간(ms)")) -> ()  [unwired: 1 out]
          n273 = local write "허가고도6 3"("허가고도") -> ()
          n274 = local write "허가고도6 2"("허가고도") -> ()
          n275 = local write "허가고도4"("허가고도") -> ()
          n276 = local write "허가고도5"("허가고도") -> ()
          n277 = local write "허가고도6"("허가고도") -> ()
          n278 = local write "허가고도7"("허가고도") -> ()
          n279 = local write "허가고도"("허가고도") -> ()
          n280 = case shown="참" "?" {
            frame False {
            }
            frame True {
              w218 = "\r"
              w225 = "\r"
              w228 = "\r"
              w233 = "\r"
              n281 = call <vilib>:"Application Directory.vi"() -> ("Application Directory"=w214:path)
              n282 = Path To String(path=w214) -> (string=w212:string)
              n283 = Concatenate Strings(w212, "\\data\\ATC app output.txt" ("문자열")) -> (w211:string)
              n284 = String To Path(string=w211) -> (path=w210:path)
              n285 = One Button Dialog(message="문서 폴더에 저장되었습니다." ("메시지")) -> ()  [unwired: 1 in, 1 out]
              n286 = Concatenate Strings("Clearance Delivery", "\r", "메모", "\r", "Ground", "\r", "메모2", w233, "Tower(Departure)", w233, "메모3", "\r", "Departure", w228, "메모 4", w228, "control", w225, "메모5", w225, "Approach", w225, "메모6", w218, "Tower(Arrival)", w218, "메모7", w218, "Ground(Arrival)", "\r", "메모8") -> (w224:string)
              n287 = Write to Text File(file (use dialog)=w210, text=w224) -> (refnum out=w243:refnum<file>, error out=w242:errorcluster)  [unwired: 2 in, 1 out]
              n288 = Close File(refnum=w243, error in=w242) -> ()  [unwired: 2 out]
            }
          }
          n289 = control-ref of="이 VI"() -> (w162:refnum<vi>)
        }
        n290 = invoke class="VI" method="FP.Close"(reference=w10) -> ()  [unwired: 2 in, 3 out]
        n291 = invoke class="VI" method="FP.Close"(reference=w9) -> ()  [unwired: 2 in, 3 out]
        n292 = while {
          tunnel: [w35] -> w5
          stop <- w36 stop-if-true
          n293 = local read "정지"() -> (w36:bool)
          n294 = event shown="[0] 키 다운" {
            selector: _ -> [_ _]
            dyn-events: _ -> [_ _]
            timeout: 0 -> [_ _]
            event Key Down {
              n295 = event-data() -> ("Char"=w40:i16)  [unwired: 1 in, 9 out]
              n296 = Equal?(x=w40, y=i16 43) -> (x = y?=w41:bool)
              n297 = case shown="참" w41 {
                frame False {
                }
                frame True {
                  n298 = call <vilib>:"Application Directory.vi"() -> ("Application Directory"=w48:path)
                  n299 = Path To String(path=w48) -> (string=w46:string)
                  n300 = Concatenate Strings(w46, "\\data\\ATC app output.txt" ("문자열")) -> (w45:string)
                  n301 = String To Path(string=w45) -> (path=w44:path)
                  n302 = Open/Create/Replace File(file path (use dialog)=w44) -> (refnum out=w69:refnum<file>, error out=w68:errorcluster)  [unwired: 5 in, 1 out]
                  n303 = Read from Text File(file (use dialog)=w69, error in=w68) -> (refnum out=w67:refnum<file>, text=w61:string, error out=w66:errorcluster)  [unwired: 2 in, 1 out]
                  n304 = Match Pattern "Clearance Delivery~Ground"(string=w61, regular expression="Clearance Delivery" ("정규식")) -> (after substring=w64:string)  [unwired: 1 in, 3 out]
                  n305 = Close File(refnum=w67, error in=w66) -> ()  [unwired: 2 out]
                  n306 = Match Pattern "Clearance Delivery~Ground"(string=w64, regular expression="Ground" ("정규식")) -> (before substring=w59:string, after substring=w60:string)  [unwired: 1 in, 2 out]
                  n307 = One Button Dialog(message="문서를 불러왔습니다." ("메시지")) -> ()  [unwired: 1 in, 1 out]
                  n308 = call <vilib>:"Trim Whitespace.vi"("string"=w59) -> ("trimmed string"=w70:string)  [unwired: 1 in]
                  n309 = Match Pattern "Tower(Departure) ~Departure"(string=w60, regular expression="Tower(Departure)" ("정규식")) -> (before substring=w58:string, after substring=w55:string)  [unwired: 1 in, 2 out]
                  n310 = local write "메모"(w70) -> ()
                  n311 = call <vilib>:"Trim Whitespace.vi"("string"=w58) -> ("trimmed string"=w71:string)  [unwired: 1 in]
                  n312 = Match Pattern "Tower(Departure) ~Departure"(string=w55, regular expression="Departure" ("정규식")) -> (before substring=w56:string, after substring=w49:string)  [unwired: 1 in, 2 out]
                  n313 = local write "메모2"(w71) -> ()
                  n314 = call <vilib>:"Trim Whitespace.vi"("string"=w56) -> ("trimmed string"=w72:string)  [unwired: 1 in]
                  n315 = Match Pattern "control~Approach"(string=w49, regular expression="control" ("정규식")) -> (before substring=w51:string, after substring=w53:string)  [unwired: 1 in, 2 out]
                  n316 = local write "메모3"(w72) -> ()
                  n317 = call <vilib>:"Trim Whitespace.vi"("string"=w51) -> ("trimmed string"=w73:string)  [unwired: 1 in]
                  n318 = Match Pattern "control~Approach"(string=w53, regular expression="Approach" ("정규식")) -> (before substring=w50:string, after substring=w76:string)  [unwired: 1 in, 2 out]
                  n319 = Match Pattern "Tower(Arrival)~Ground(Arrival)"(string=w76, regular expression="Tower(Arrival)" ("정규식")) -> (before substring=w78:string, after substring=w80:string)  [unwired: 1 in, 2 out]
                  n320 = local write "메모 4"(w73) -> ()
                  n321 = call <vilib>:"Trim Whitespace.vi"("string"=w50) -> ("trimmed string"=w74:string)  [unwired: 1 in]
                  n322 = Match Pattern "Tower(Arrival)~Ground(Arrival)"(string=w80, regular expression="Ground(Arrival)" ("정규식")) -> (before substring=w81:string, after substring=w82:string)  [unwired: 1 in, 2 out]
                  n323 = local write "메모6"(w78) -> ()
                  n324 = local write "메모5"(w74) -> ()
                  n325 = local write "메모7"(w81) -> ()
                  n326 = local write "메모8"(w82) -> ()
                }
              }
              n327 = Equal?(x=w40, y=i16 45) -> (x = y?=w43:bool)
              n328 = case shown="참" w43 {
                frame False {
                }
                frame True {
                  w91 = "\r"
                  w103 = "\r"
                  w105 = "\r"
                  w108 = "\r"
                  n329 = local read "메모6"() -> (w94:string)
                  n330 = local read "메모5"() -> (w95:string)
                  n331 = local read "메모 4"() -> (w96:string)
                  n332 = local read "메모7"() -> (w92:string)
                  n333 = local read "메모2"() -> (w98:string)
                  n334 = local read "메모3"() -> (w97:string)
                  n335 = local read "메모"() -> (w99:string)
                  n336 = local read "메모8"() -> (w88:string)
                  n337 = One Button Dialog(message="문서 폴더에 저장되었습니다." ("메시지")) -> ()  [unwired: 1 in, 1 out]
                  n338 = call <vilib>:"Application Directory.vi"() -> ("Application Directory"=w87:path)
                  n339 = Path To String(path=w87) -> (string=w85:string)
                  n340 = Concatenate Strings(w85, "\\data\\ATC app output.txt" ("문자열")) -> (w84:string)
                  n341 = String To Path(string=w84) -> (path=w83:path)
                  n342 = Concatenate Strings("Clearance Delivery", "\r", w99, "\r", "Ground", "\r", w98, w108, "Tower(Departure)", w108, w97, "\r", "Departure", w105, w96, w105, "control", w103, w95, w103, "Approach", w103, w94, w91, "Tower(Arrival)", w91, w92, w91, " Ground(Arrival)", "\r", w88) -> (w102:string)
                  n343 = Write to Text File(file (use dialog)=w83, text=w102) -> (refnum out=w116:refnum<file>, error out=w115:errorcluster)  [unwired: 2 in, 1 out]
                  n344 = Close File(refnum=w116, error in=w115) -> ()  [unwired: 2 out]
                }
              }
            }
            event Timeout {
              n345 = event-data() -> ()  [unwired: 1 in, 3 out]
            }
          }
          n346 = control-ref of="이 VI"() -> (w35:refnum<vi>)
          n347 = Wait (ms)(milliseconds to wait=u32 800 ("대기 시간(ms)")) -> ()  [unwired: 1 out]
        }
        n348 = invoke class="VI" method="FP.Close"(reference=w7) -> ()  [unwired: 2 in, 3 out]
        n349 = invoke class="VI" method="FP.Close"(reference=w6) -> ()  [unwired: 2 in, 3 out]
        n350 = control-ref of="이 VI"() -> (w3:refnum<vi>)
        n351 = invoke class="VI" method="FP.Close"(reference=w5) -> ()  [unwired: 2 in, 3 out]
      }
      n352 = invoke class="VI" method="FP.Close"(reference=w2) -> ()  [unwired: 2 in, 3 out]
    }
  }
